vi "CCExcelToDcmStoreScuCallback.vi"(4 "Callback Str":refnum<vi>, 5 "Event Data":T1, 6 "Control Ref":refnum<k24>, 7 "Event Common Data":T2) -> ()   [LabVIEW 2013, in "Medimatic.lvlib"]
uses:
  Medimatic.lvlib
  C:/Users/Simon/SkyDrive/LabView/2013/DM2020/DICOM/ClearCanvasNewBuild/ClearCanvas.Dicom.dll
  ClearCanvasNewBuild/ClearCanvas.Dicom.dll
  C:/Program Files (x86)/National Instruments/LabVIEW 2011/examples/comm/dotnet/EventExample.dll
  Program Files (x86)/National Instruments/LabVIEW 2011/examples/comm/dotnet/EventExample.dll
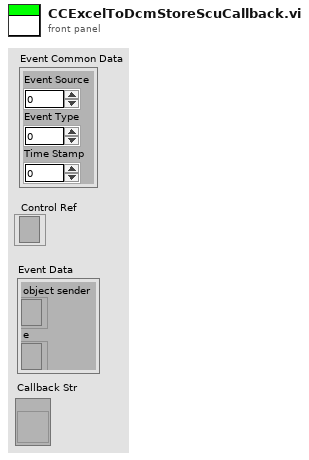
[diagram p1: front panel]
types:
  T1 = cluster{"object sender":refnum<k24>, "e":refnum<k24>}
  T2 = cluster{"Event Source":i32, "Event Type":u32, "Time Stamp":u32}
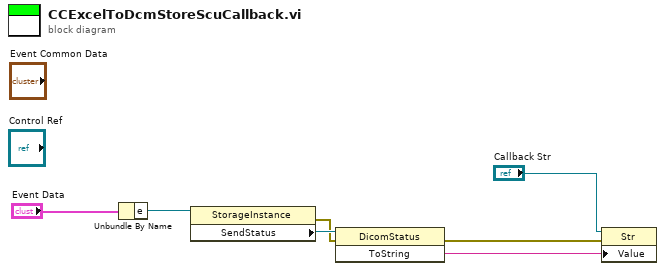
[diagram p0: block diagram]
diagram:
  n1 = Unbundle By Name("Event Data") -> ("e"=w6:refnum<k24>)
  n2 = property class="StorageInstance"(reference=w6) -> (error out=w4:errorcluster, "SendStatus"=w5:refnum<k24>)  [unwired: 1 in, 1 out]
  n3 = invoke class="DicomStatus" method="ToString"(reference=w5, error in=w4) -> (error out=w2:errorcluster, "ToString"=w3:string)  [unwired: 1 in, 1 out]
  n4 = property class="Str"(reference="Callback Str", error in=w2, "Value"=w3) -> ()  [unwired: 2 out]
